vi "SetDownsample.vi"(9 "Downsample rate":i32, 11 "scope in":T1={"scope mode"=enum."Stopped", "ticker"=refnum, "samples per simulated"=0, "FPGA ref"=refnum, "P2P params"={"instrument handle"="", "stream session"=refnum, "scale"={"offset"=0.0, "gain"=0.0, "reserved 1"=0.0, "reserved 2"=0.0}, "actual sample rate"=10000000.0, "Trigger"=enum."PFI 0", "SCOPE Resource"="Dev1", "input impedance"=0}, "data mode"=enum."Real IO"} {"P2P params"."input impedance" items=["1 mega ohm"=0, "50 ohms"=2]; "P2P params"."actual sample rate" format="%.2p"}) -> (3 "scope out":T1={"scope mode"=enum."Stopped", "ticker"=refnum, "samples per simulated"=0, "FPGA ref"=refnum, "P2P params"={"instrument handle"="", "stream session"=refnum, "scale"={"offset"=0.0, "gain"=0.0, "reserved 1"=0.0, "reserved 2"=0.0}, "actual sample rate"=10000000.0, "Trigger"=enum."PFI 0", "SCOPE Resource"="Dev1", "input impedance"=0}, "data mode"=enum."Real IO"} {"P2P params"."input impedance" items=["1 mega ohm"=0, "50 ohms"=2]; "P2P params"."actual sample rate" format="%.2p"})   [LabVIEW 2013]
uses:
  controls/scope_params.ctl
  Utilities/Ticker/Ticker.lvclass
  controls/ScopeMode.ctl
  Config/FPGAref.ctl
  P2P streaming/P2P params.ctl
  P2P streaming/trigger_source.ctl
  FPGA/DataMode.ctl
  <vilib>/rvi/interface/common/niFpgaWaitOnOcc.vi
  <vilib>/Utility/error.llb/Error Cluster From Error Code.vi
  <vilib>/rvi/errors/niLvFpgaAdjustHostInterfaceError.vi
  <vilib>/rvi/interface/nirviReadWriteControl/nirviReadWriteControl.xnode
  NiFpgaLv.dll
  <vilib>/rvi/interface/Simulation/niFpgaSimulationCallBeginRW.vi
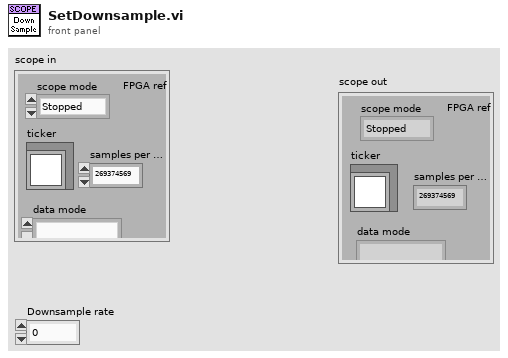
[diagram p1: front panel]
types:
  T1 = typedef "scope_params.ctl" = cluster{"scope mode":T2, "ticker":refnum<class "Ticker.lvclass">, "samples per simulated":u32, "FPGA ref":T3, "P2P params":T4, "data mode":T6}
  T2 = typedef "ScopeMode.ctl" = enum16{"Stopped", "Single", "Running"}
  T3 = typedef "FPGAref.ctl" = refnum<k20>
  T4 = typedef "P2P params.ctl" = cluster{"instrument handle":refnum<k15>, "stream session":refnum<k20>, "scale":cluster{"offset":dbl, "gain":dbl, "reserved 1":dbl, "reserved 2":dbl}, "actual sample rate":dbl, "Trigger":T5, "SCOPE Resource":refnum<k15>, "input impedance":u32}
  T5 = typedef "trigger_source.ctl" = enum16{"PFI 0", "PFI 1", "Software"}
  T6 = typedef "DataMode.ctl" = enum16{"Real IO", "Simulated"}
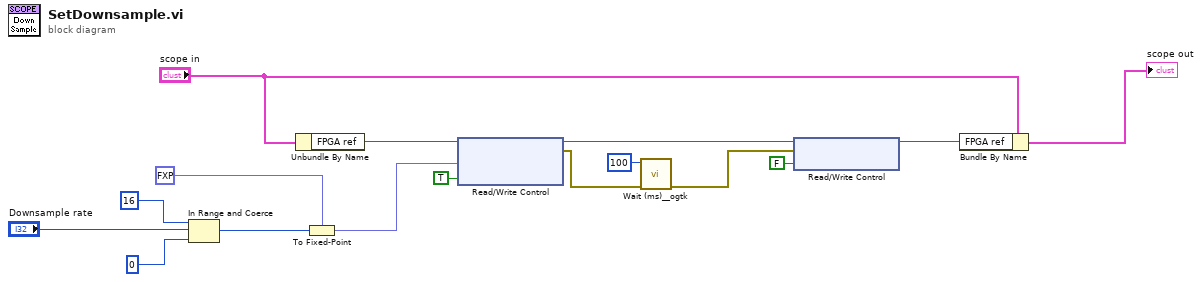
[diagram p0: block diagram]
diagram:
  n1 = In Range and Coerce(upper limit=16 ("lower limit"), x="Downsample rate", lower limit=0) -> ()  [unwired: 2 out]
  n2 = Unbundle By Name("scope in") -> ("FPGA ref"=w15:T3)
  n3 = To Fixed-Point(fixed-point type=fxp<+,8,8> 0.0 ("Downsample"), number="Downsample rate") -> (fixed-point=w13:fxp<+,8,8>)
  n4 = xnode "Read/Write Control"("FPGA VI Reference In"=w15, "Downsample"=w13, "Set downsample"=TRUE) -> ("FPGA VI Reference Out"=w9:T3, "error out"=w8:errorcluster)  [unwired: 1 in]
  n5 = call <userlib>:"Wait (ms)__ogtk.vi"("error in (no error)"=w8, "milliseconds to wait"=u32 100) -> ("error out"=w6:errorcluster)  [unwired: 8 in, 1 out]
  n6 = xnode "Read/Write Control"("FPGA VI Reference In"=w9, "error in"=w6, "Set downsample"=FALSE) -> ("FPGA VI Reference Out"=w2:T3)  [unwired: 1 out]
  n7 = Bundle By Name(cluster="scope in", "FPGA ref"=w2) -> (→"scope out":T1)
